vi "set interation log.vi"(8 "error in (no error)":errorcluster, 11 "iter":i32) -> (0 "error out":errorcluster)   [LabVIEW 2019, in "libSimulationControl.lvlib"]
doc: "void set_interation_log(int iter);"
uses:
  libSimulationControl.lvlib
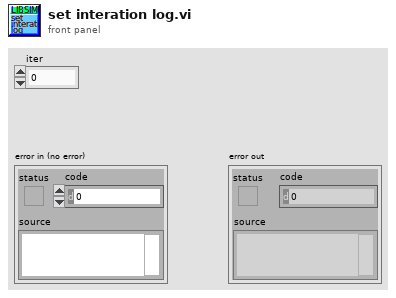
[diagram p1: front panel]
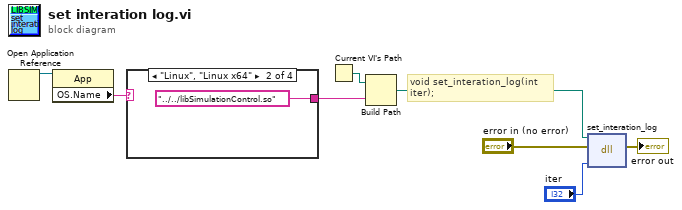
[diagram p0: block diagram]
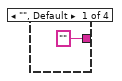
[diagram p2: hidden frame]
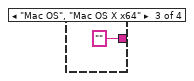
[diagram p3: hidden frame]
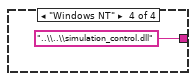
[diagram p4: hidden frame]
diagram:
  # "void set_interation_log(int iter);"
  n1 = Open Application Reference() -> (3:w3:refnum<vi>)  [unwired: 4 in, 1 out]
  n2 = property class="App"(reference=w3) -> ("OS.Name"=w2:string)  [unwired: 1 in, 2 out]
  n3 = case shown="\"Linux\", \"Linux x64\"" w2 {
    tunnel: ["" ("return type") "../../libSimulationControl.so" ("name or relative path") "" ("return type") "..\\..\\simulation_control.dll" ("name or relative path")] -> w1
    frame "", Default {
    }
    frame "Linux", "Linux x64" {
    }
    frame "Mac OS", "Mac OS X x64" {
    }
    frame "Windows NT" {
    }
  }
  n4 = Current VI's Path() -> (path=w5:path)
  n5 = Build Path(base path=w5, name or relative path=w1) -> (appended path=w4:path)
  n6 = dll-call lib="home/paul/Schreibtisch/Biogas_plant_setup/LabView/lib/libSimulationControl/libSimulationControl.*" fn="set_interation_log"(path in=w4, error in="error in (no error)", "iter"="iter") -> (error out=→"error out":errorcluster)  [unwired: 3 in, 1 out]
